vi "CR-Initial CameraCCD12.vi"(8 "error in (no error)":errorcluster caption="错误输入（无错误）") -> (0 "error out":errorcluster caption="错误输出", 2 "Session Out 2":T1 caption="Session Out", 3 "Session Out":T1)   [LabVIEW 2017]
uses:
  <vilib>/userdefined/High Color/IMAQdx.ctl
  <vilib>/vision/driver/IMAQdx.llb/IMAQdx Acquisition Mode.ctl
  <vilib>/vision/driver/NI_Vision_Acquisition_Software.lvlib
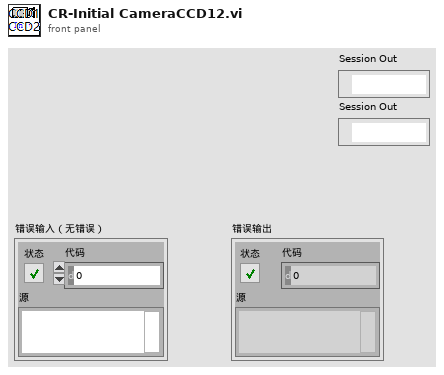
[diagram p1: front panel]
types:
  T1 = typedef "IMAQdx.ctl" = refnum<k21>
  T2 = typedef "NI_Vision_Acquisition_Software.lvlib/IMAQdx Acquisition Mode.ctl" = enum32{"One Shot", "Continuous"}
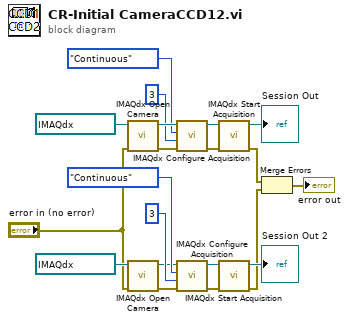
[diagram p0: block diagram]
diagram:
  n1 = call <vilib>:"IMAQdx Open Camera.vi"("error in"="error in (no error)", "Session In"=T1 "cam2") -> ("error out"=w17:errorcluster, "Session Out"=w20:T1)  [unwired: 8 in]
  n2 = call <vilib>:"IMAQdx Open Camera.vi"("error in"="error in (no error)", "Session In"=T1 "cam3") -> ("error out"=w14:errorcluster, "Session Out"=w11:T1)  [unwired: 8 in]
  n3 = call <vilib>:"IMAQdx Configure Acquisition.vi"("error in"=w17, "Number of Buffers"=u32 3, "Continuous?"=IMAQdx_Acquisition_Mode."Continuous", "Session In"=w20) -> ("error out"=w7:errorcluster, "Session Out"=w8:T1)  [unwired: 6 in]
  n4 = call <vilib>:"IMAQdx Configure Acquisition.vi"("error in"=w14, "Number of Buffers"=u32 3, "Continuous?"=IMAQdx_Acquisition_Mode."Continuous", "Session In"=w11) -> ("error out"=w2:errorcluster, "Session Out"=w4:T1)  [unwired: 6 in]
  n5 = call <vilib>:"IMAQdx Start Acquisition.vi"("error in"=w7, "Session In"=w8) -> ("error out"=w5:errorcluster, "Session Out"=→"Session Out":T1)  [unwired: 8 out]
  n6 = call <vilib>:"IMAQdx Start Acquisition.vi"("error in"=w2, "Session In"=w4) -> ("error out"=w1:errorcluster, "Session Out"=→"Session Out 2":T1)  [unwired: 8 out]
  n7 = Merge Errors(w5, w1) -> (→"error out":errorcluster)
